vi "Pre Launch Init.vi"(11 "ErrorHanlder in":refnum<class "ErrorHanlder.lvclass"> caption="操作者输入") -> (0 "error out":errorcluster caption="错误输出", 3 "ErrorHanlder out":refnum<class "ErrorHanlder.lvclass"> caption="操作者输出")   [LabVIEW 2019, in "ErrorHanlder.lvlib" / "ErrorHanlder.lvclass"]
doc: "(<B>文件名</B>: Actor Framework.lvlib:Actor.lvclass:Pre Launch Init.vi)\n\n定义启动嵌套操作者方法被调用之后、操作者核心方法开始运行之前的操作。\n\n默认情况下，该方法不执行任何操作。子孙类重写该方法定义具体的操作。"
uses:
  ErrorHanlder.lvclass
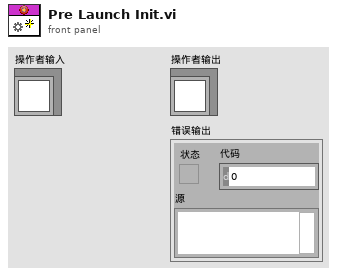
[diagram p1: front panel]
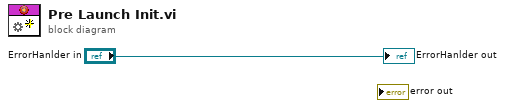
[diagram p0: block diagram]
diagram:
  "ErrorHanlder out" <- "ErrorHanlder in"
